vi "Trabalho no5.vi"() -> ()   [LabVIEW 2017]
panel:
  out "Status do controlador":bool[](array[boolean])
  out "Modo de operação":string
  out "Perfil de funcionamento":u8(ring) items=["Off"=0, "Confort"=1, "Standby"=2, "Night"=4]
  out "String 2":string
  out "String":string
  in  "STOP":bool
  in  "Array":dbl
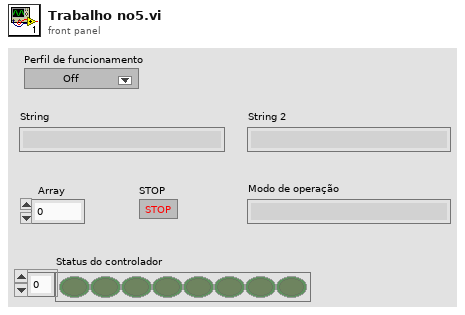
[diagram p1: front panel]
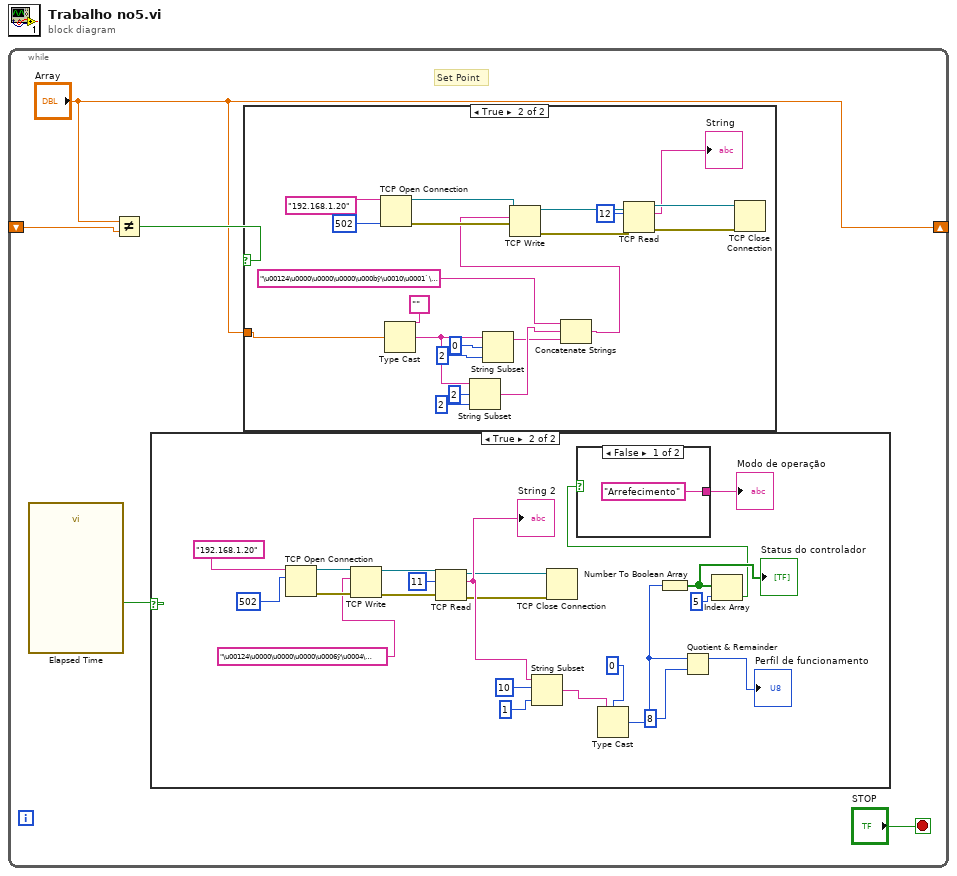
[diagram p0: block diagram]
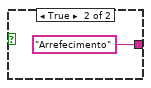
[diagram p3: hidden frame]
diagram:
  n1 = while {
    shift-right: ["Array"] -> _
    shift-left: _ -> [w2]
    stop <- "STOP" stop-if-true
    # "Set Point"
    n2 = call "Elapsed Time"() -> ("Time has Elapsed"=w1:bool)  [unwired: 12 in, 7 out]
    n3 = Not Equal?(x="Array", y=w2) -> (x != y?=w4:bool)
    n4 = case shown="True" w1 {
      frame False {
      }
      frame True {
        n5 = TCP Open Connection(address="192.168.1.20", remote port or service name=u16 502) -> (connection ID=w17:refnum<k5>, error out=w20:errorcluster)  [unwired: 3 in]
        n6 = TCP Write(connection ID=w17, data in="\u00124\u0000\u0000\u0000\u0006ÿ\u0004\u0001\u0005\u0000\u0001", error in (no error)=w20) -> (connection ID out=w18:refnum<k5>, error out=w21:errorcluster)  [unwired: 1 in, 1 out]
        n7 = TCP Read(connection ID=w18, bytes to read=11, error in (no error)=w21) -> (connection ID out=w19:refnum<k5>, data out=w23:string, error out=w22:errorcluster)  [unwired: 2 in]
        "String 2" <- w23
        n8 = String Subset(string=w23, offset (0)=10, length (rest)=1 ("length (rest)")) -> (substring=w24:string)
        n9 = TCP Close Connection(connection ID=w19, error in (no error)=w22) -> ()  [unwired: 1 in, 2 out]
        n10 = Type Cast(type=u8 0, x=w24) -> (*(type *) &x=w26:u8)
        n11 = Number To Boolean Array(number=w26) -> (Boolean array=w27:bool[])
        "Status do controlador" <- w27
        n12 = Quotient & Remainder(x=w26, y=u8 8) -> (x-y*floor(x/y)=→"Perfil de funcionamento":u8)  [unwired: 1 out]
        n13 = Index Array(array=w27, index=5) -> (element=w8:bool)
        n14 = case shown="False" w8 {
          tunnel: ["Arrefecimento" "Arrefecimento"] -> w10
          frame False {
          }
          frame True {
          }
        }
        "Modo de operação" <- w10
      }
    }
    n15 = case shown="True" w4 {
      tunnel: "Array" -> [_ w30]
      frame False {
      }
      frame True {
        n16 = TCP Open Connection(address="192.168.1.20", remote port or service name=u16 502) -> (connection ID=w50:refnum<k5>, error out=w47:errorcluster)  [unwired: 3 in]
        n17 = Type Cast(type="", x=w30) -> (*(type *) &x=w37:string)
        n18 = String Subset(string=w37, offset (0)=2, length (rest)=2 ("length (rest)")) -> (substring=w36:string)
        n19 = String Subset(string=w37, offset (0)=0, length (rest)=2 ("length (rest)")) -> (substring=w35:string)
        n20 = Concatenate Strings("\u00124\u0000\u0000\u0000\u000bÿ\u0010\u0001`\u0000\u0002\u0004", w36, w35) -> (w40:string)
        n21 = TCP Write(connection ID=w50, data in=w40, error in (no error)=w47) -> (connection ID out=w49:refnum<k5>, error out=w46:errorcluster)  [unwired: 1 in, 1 out]
        n22 = TCP Read(connection ID=w49, bytes to read=12, error in (no error)=w46) -> (connection ID out=w48:refnum<k5>, data out=→"String":string, error out=w45:errorcluster)  [unwired: 2 in]
        n23 = TCP Close Connection(connection ID=w48, error in (no error)=w45) -> ()  [unwired: 1 in, 2 out]
      }
    }
  }
